vi "ABCThirdKicker.vi"(6 "Tactic index in":i32, 7 "first call":bool, 8 "error in (no error) 2":errorcluster, 10 "Game in":refnum<class "Game.lvclass">, 11 "ABCThirdKicker in":refnum<class "ABCThirdKicker.lvclass">) -> (0 "error out 2":errorcluster, 1 "tactic index":i32, 2 "Robot out":refnum<class "Robot.lvclass">, 3 "ABCThirdKicker out":refnum<class "ABCThirdKicker.lvclass">)   [LabVIEW 2023, in "ABCThirdKicker.lvclass"]
uses:
  ABCThirdKicker.lvclass
  C:/Users/ebert/Desktop/roboime/SSL_AI/Role_class/Role.lvclass
  Game_class/Game.lvclass
  Robot_class/Robot.lvclass
  Role_class/Role.lvclass/Role.ctl
  Tacticbook_class/Tacticbook.lvclass/Tacticbook.ctl
  HaltTactic_class/HaltTactic.lvclass/HaltTactic.ctl
  ShootTactic_class/States.ctl
  ShootTactic_class/ShootTactic.lvclass/ShootTactic.ctl
  Tacticbook_class/Read HaltTactic.vi
  HaltTactic_class/Read States.vi
  Tacticbook_class/Write HaltTactic.vi
  Tacticbook_class/Read WaitPassTactic.vi
  Tacticbook_class/Write WaitPassTactic.vi
  Tacticbook_class/Read ShootTactic.vi
  ShootTactic_class/Read States.vi
  Tacticbook_class/Write ShootTactic.vi
  Role_class/Read Tacticbook.vi
  Role_class/Write Tacticbook.vi
  Role_class/Write tactic_index.vi
  Role_class/Read RobotRef.vi
  Tacticbook_class/Tacticbook.lvclass
  HaltTactic_class/HaltTactic.lvclass
  WaitPassTactic_class/WaitPassTactic.lvclass
  ShootTactic_class/ShootTactic.lvclass
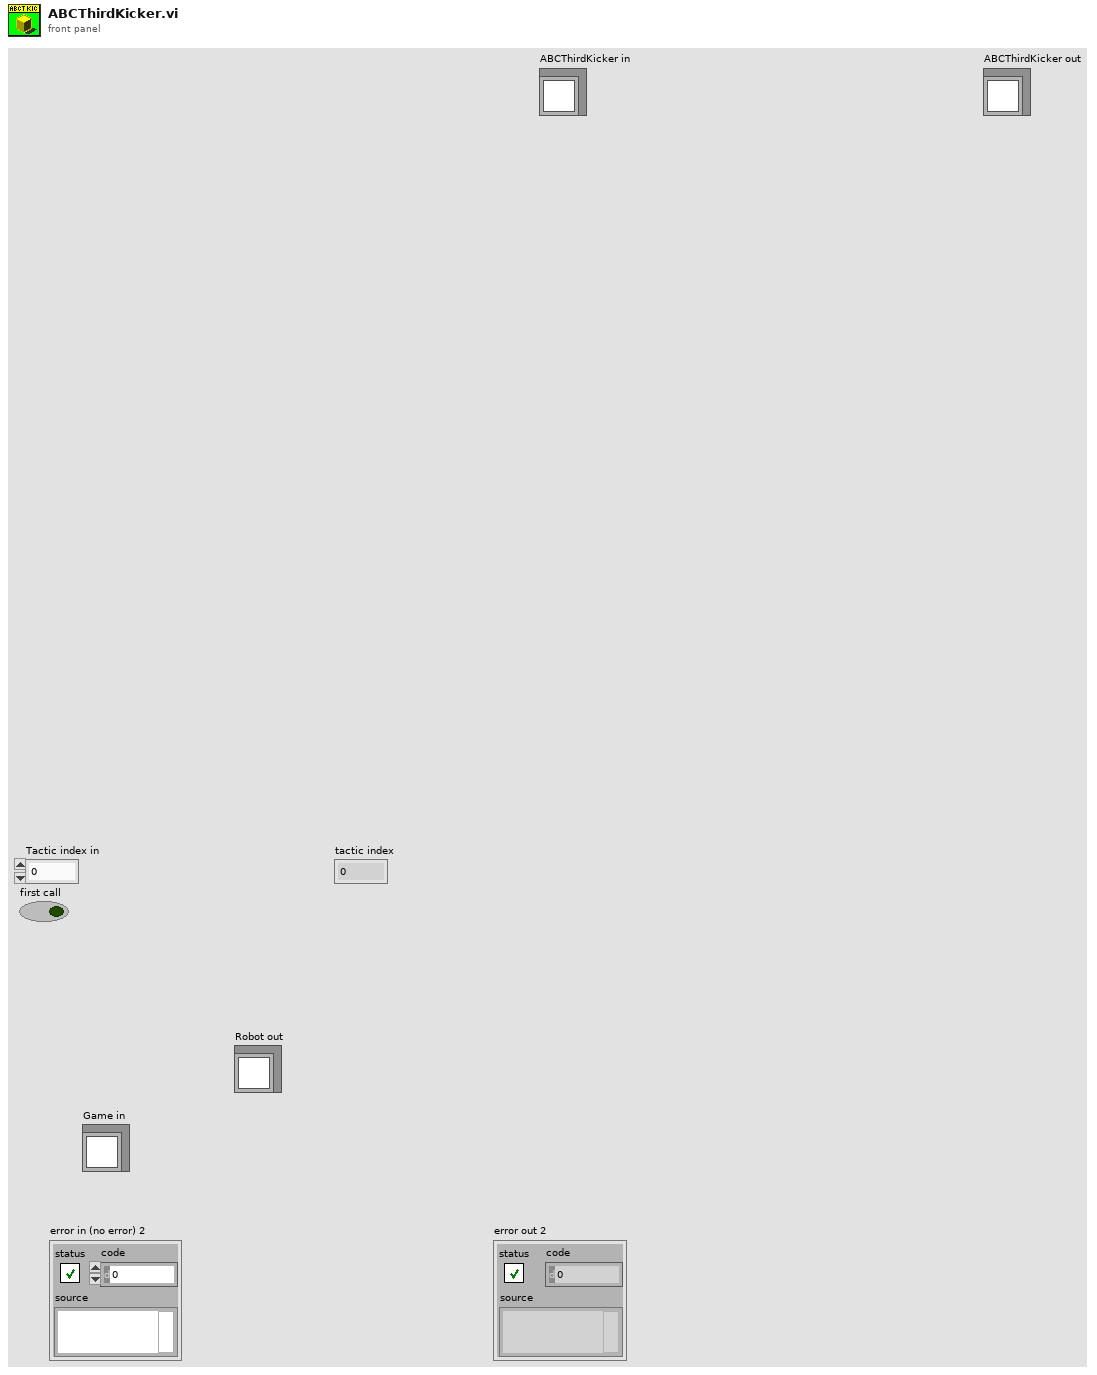
[diagram p1: front panel]
types:
  T1 = typedef "ShootTactic.lvclass/States.ctl" = enum16{"BallInGoalieArea", "Exit", "KickToGoal", "StealBall"}
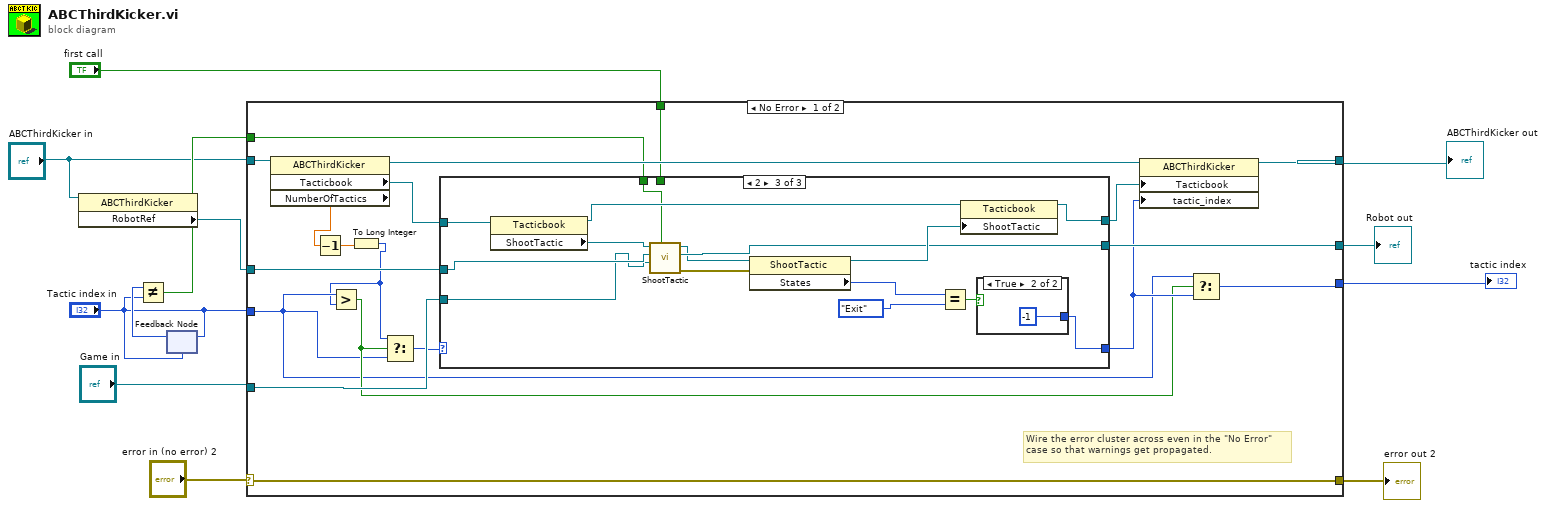
[diagram p0: block diagram]
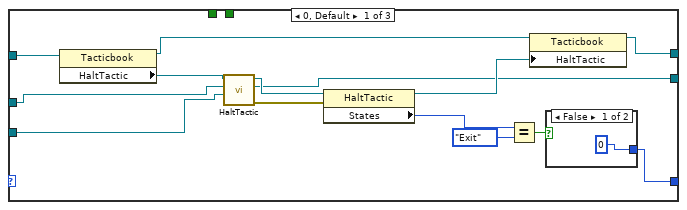
[diagram p2: hidden frame]
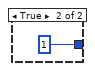
[diagram p3: hidden frame]
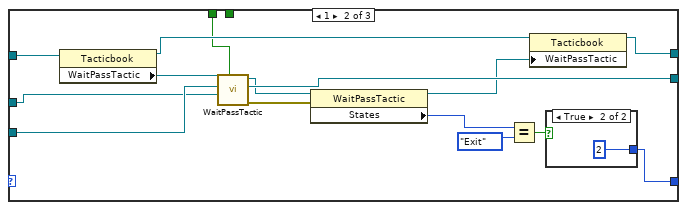
[diagram p4: hidden frame]
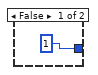
[diagram p5: hidden frame]
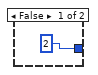
[diagram p6: hidden frame]
diagram:
  n1 = property class="ABCThirdKicker"(reference="ABCThirdKicker in") -> ("RobotRef"=w10:refnum<class "Robot.lvclass">)  [unwired: 1 in, 2 out]
  n2 = feedback #1("Tactic index in") -> (w6:i32)
  n3 = Not Equal?(x=w6, y="Tactic index in") -> (x != y?=w4:bool)
  n4 = feedback-in #1("Tactic index in") -> ()
  n5 = case shown="No Error" "error in (no error) 2" {
    selector: "error in (no error) 2" -> [w31 w84]
    tunnel: [w31 w84] -> w11
    tunnel: [w29 w83] -> w1
    tunnel: "ABCThirdKicker in" -> [w30 w83]
    tunnel: w10 -> [w26 w82]
    tunnel: [w25 w82] -> w3
    tunnel: "Game in" -> [w23 _]
    tunnel: [w21 _] -> w9
    tunnel: "Tactic index in" -> [w18 _]
    tunnel: "first call" -> [w16 _]
    tunnel: w4 -> [w13 _]
    frame No Error {
      # "Wire the error cluster across even in the \"No Error\"\ncase so that warnings get propagated."
      n6 = property class="ABCThirdKicker"(reference=w30) -> (reference out=w28:refnum<class "ABCThirdKicker.lvclass">, "Tacticbook"=w27:refnum<class "Tacticbook.lvclass">, "NumberOfTactics"=w17:dbl)  [unwired: 1 in, 1 out]
      n7 = Decrement(x=w17) -> (x-1=w15:dbl)
      n8 = To Long Integer(number=w15) -> (32bit integer=w14:i32)
      n9 = Greater?(x=w18, y=w14) -> (0:w19:bool)
      n10 = Select(t=w14, s=w19, f=w18) -> (s? t:f=w20:i32)
      n11 = case shown="2" w20 {
        tunnel: [w39 w50 w73] -> w22
        tunnel: w27 -> [w45 w62 w79]
        tunnel: w26 -> [w37 w53 w71]
        tunnel: [w34 w61 w69] -> w25
        tunnel: [w42 w57 w76] -> w24
        tunnel: w23 -> [w36 w54 w70]
        tunnel: w16 -> [_ _ _]
        tunnel: w13 -> [_ w49 w65]
        frame 0, Default {
          n12 = property class="Tacticbook"(reference=w45) -> (reference out=w44:refnum<class "Tacticbook.lvclass">, "HaltTactic"=w38:refnum<class "HaltTactic.lvclass">)  [unwired: 1 in, 1 out]
          n13 = call-dynamic "HaltTactic.vi"("Game in"=w36, "Robot"=w37, "HaltTactic in"=w38) -> ("error out"=w33:errorcluster, "Robot out"=w34:refnum<class "Robot.lvclass">, "HaltTactic out"=w35:refnum<class "HaltTactic.lvclass">)  [unwired: 6 in]
          n14 = property class="HaltTactic"(reference=w35, error in=w33) -> (reference out=w43:refnum<class "HaltTactic.lvclass">, "States"=w40:enum16{"Halt", "Exit"})  [unwired: 1 out]
          n15 = Equal?(x=w40, y=enum16{"Halt", "Exit"}."Exit") -> (x = y?=w41:bool)
          n16 = property class="Tacticbook"(reference=w44, "HaltTactic"=w43) -> (reference out=w42:refnum<class "Tacticbook.lvclass">)  [unwired: 1 in, 1 out]
          n17 = case shown="False" w41 {
            tunnel: [0 1] -> w39
            frame False {
            }
            frame True {
            }
          }
        }
        frame 1 {
          n18 = property class="Tacticbook"(reference=w62) -> (reference out=w59:refnum<class "Tacticbook.lvclass">, "WaitPassTactic"=w56:refnum<class "WaitPassTactic.lvclass">)  [unwired: 1 in, 1 out]
          n19 = call-dynamic "WaitPassTactic.vi"("first call"=w49, "Robot"=w53, "Game in"=w54, "WaitPassTactic in"=w56) -> ("error out"=w60:errorcluster, "Robot out"=w61:refnum<class "Robot.lvclass">, "WaitPassTactic out"=w55:refnum<class "WaitPassTactic.lvclass">)  [unwired: 5 in]
          n20 = property class="WaitPassTactic"(reference=w55, error in=w60) -> (reference out=w58:refnum<class "WaitPassTactic.lvclass">, "States"=w51:enum16{"State 0", "State 1", "State 2", "Exit"})  [unwired: 1 out]
          n21 = Equal?(x=w51, y=enum16{"State 0", "State 1", "State 2", "Exit"}."Exit") -> (x = y?=w52:bool)
          n22 = property class="Tacticbook"(reference=w59, "WaitPassTactic"=w58) -> (reference out=w57:refnum<class "Tacticbook.lvclass">)  [unwired: 1 in, 1 out]
          n23 = case shown="True" w52 {
            tunnel: [1 2] -> w50
            frame False {
            }
            frame True {
            }
          }
        }
        frame 2 {
          n24 = property class="Tacticbook"(reference=w79) -> (reference out=w78:refnum<class "Tacticbook.lvclass">, "ShootTactic"=w72:refnum<class "ShootTactic.lvclass">)  [unwired: 1 in, 1 out]
          n25 = call "ShootTactic.vi"("firstCall?"=w65, "Game in"=w70, "Robot"=w71, "ShootTactic in"=w72) -> ("error out"=w67:errorcluster, "Robot out"=w69:refnum<class "Robot.lvclass">, "ShootTactic out"=w68:refnum<class "ShootTactic.lvclass">)  [unwired: 4 in, 1 out]
          n26 = property class="ShootTactic"(reference=w68, error in=w67) -> (reference out=w77:refnum<class "ShootTactic.lvclass">, "States"=w74:T1)  [unwired: 1 out]
          n27 = Equal?(x=w74, y=States."Exit") -> (x = y?=w75:bool)
          n28 = property class="Tacticbook"(reference=w78, "ShootTactic"=w77) -> (reference out=w76:refnum<class "Tacticbook.lvclass">)  [unwired: 1 in, 1 out]
          n29 = case shown="True" w75 {
            tunnel: [2 -1] -> w73
            frame False {
            }
            frame True {
            }
          }
        }
      }
      n30 = property class="ABCThirdKicker"(reference=w28, "Tacticbook"=w24, "tactic_index"=w22) -> (reference out=w29:refnum<class "ABCThirdKicker.lvclass">)  [unwired: 1 in, 1 out]
      n31 = Select(t=w18, s=w19, f=w22) -> (s? t:f=w21:i32)
    }
    frame Error {
    }
  }
  "ABCThirdKicker out" <- w1
  "error out 2" <- w11
  "tactic index" <- w9
  "Robot out" <- w3
